vi "SLSC Error Suppression.vi"(3 "error in (no error)":errorcluster, 4 "Popup Error?":bool, 5 "Clear All Error?":bool) -> (6 "error?":bool, 10 "error out":errorcluster)   [LabVIEW 2015, in "SLSC CD Shared.lvlib"]
uses:
  SLSC CD Shared.lvlib
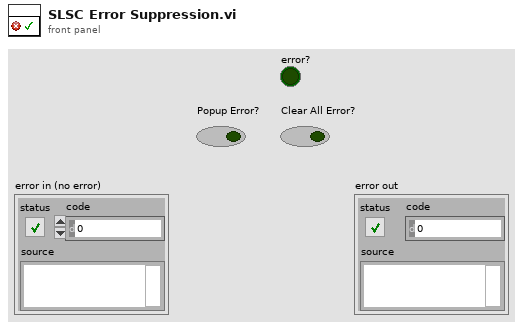
[diagram p1: front panel]
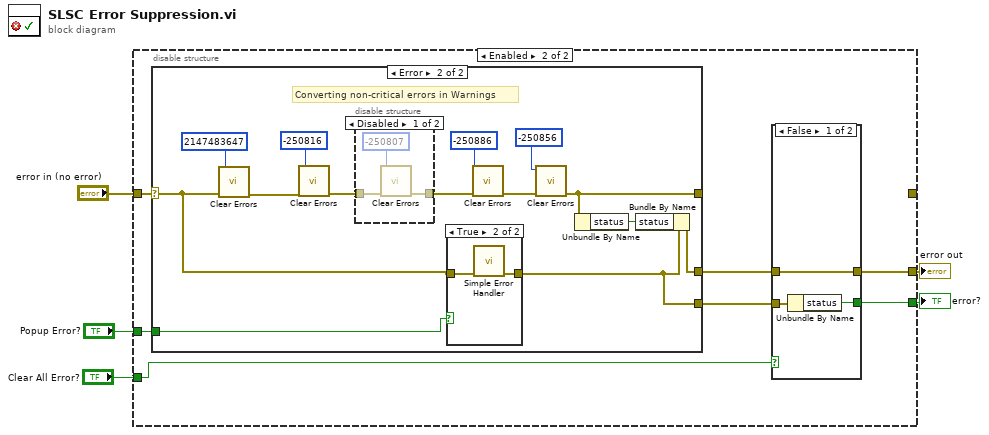
[diagram p0: block diagram]
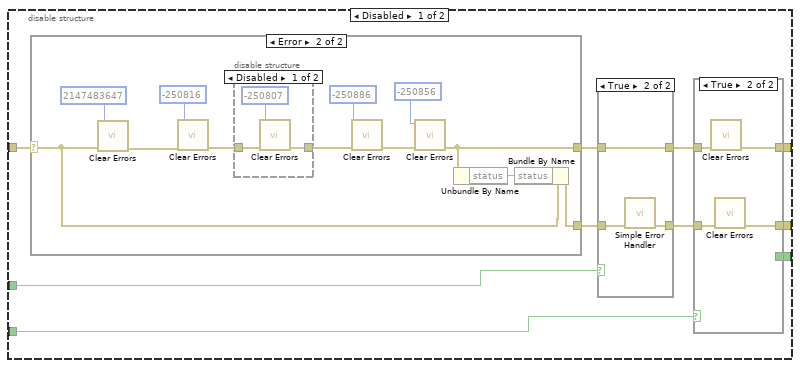
[diagram p2: hidden frame]
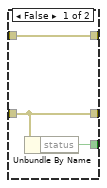
[diagram p3: hidden frame]
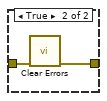
[diagram p7: hidden frame]
diagram:
  n1 = disable-structure shown="Enabled" {
    disable-tunnel: "error in (no error)" -> [w15 w51]
    disable-tunnel: "Popup Error?" -> [w14 w46]
    disable-tunnel: [w12 w49] -> w3
    disable-tunnel: [w9 _] -> _
    disable-tunnel: "Clear All Error?" -> [w8 w47]
    disable-tunnel: [w6 w48] -> w1
    frame Disabled {
      n2 = case shown="Error" w15 {
        selector: w15 -> [w28 w29]
        tunnel: [w28 w32] -> w11
        tunnel: [w28 w30] -> w7
        frame No Error {
        }
        frame Error {
          n3 = call <vilib>:"Clear Errors.vi"("error in (no error)"=w29, "specific error code to clear (0: all)"=2147483647) -> ("error out"=w33:errorcluster)  [unwired: 4 in, 1 out]
          n4 = call <vilib>:"Clear Errors.vi"("error in (no error)"=w33, "specific error code to clear (0: all)"=-250816) -> ("error out"=w39:errorcluster)  [unwired: 4 in, 1 out]
          n5 = disable-structure shown="Disabled" {
            disable-tunnel: w39 -> [w42 w44]
            disable-tunnel: [w41 w44] -> w40
            frame Disabled {
              n6 = call <vilib>:"Clear Errors.vi"("error in (no error)"=w42, "specific error code to clear (0: all)"=-250807) -> ("error out"=w41:errorcluster)  [unwired: 4 in, 1 out]
            }
            frame Enabled {
            }
          }
          n7 = call <vilib>:"Clear Errors.vi"("error in (no error)"=w40, "specific error code to clear (0: all)"=-250886) -> ("error out"=w36:errorcluster)  [unwired: 4 in, 1 out]
          n8 = call <vilib>:"Clear Errors.vi"("error in (no error)"=w36, "specific error code to clear (0: all)"=-250856) -> ("error out"=w32:errorcluster)  [unwired: 4 in, 1 out]
          n9 = Unbundle By Name(w32) -> ("status"=w31:bool)
          n10 = Bundle By Name(cluster=w29, "status"=w31) -> (w30:errorcluster)
        }
      }
      n11 = case shown="True" w14 {
        tunnel: w7 -> [w24 w27]
        tunnel: [w24 w26] -> w13
        tunnel: [w23 w25] -> w10
        tunnel: w11 -> [w23 w25]
        frame False {
        }
        frame True {
          n12 = call <vilib>:"Simple Error Handler.vi"("error in (no error)"=w27) -> ("error out"=w26:errorcluster)  [unwired: 4 in, 4 out]
        }
      }
      n13 = case shown="True" w8 {
        tunnel: w13 -> [w17 w22]
        tunnel: [w17 w21] -> w12
        tunnel: w10 -> [w18 w20]
        tunnel: [w18 w19] -> w9
        tunnel: [w16 _] -> w6
        frame False {
          n14 = Unbundle By Name(w17) -> ("status"=w16:bool)
        }
        frame True {
          n15 = call <vilib>:"Clear Errors.vi"("error in (no error)"=w20) -> ("error out"=w19:errorcluster)  [unwired: 5 in, 1 out]
          n16 = call <vilib>:"Clear Errors.vi"("error in (no error)"=w22) -> ("error out"=w21:errorcluster)  [unwired: 5 in, 1 out]
        }
      }
    }
    frame Enabled {
      n17 = case shown="Error" w51 {
        selector: w51 -> [w57 w60]
        tunnel: [w57 w63] -> _
        tunnel: [w57 w61] -> w50
        tunnel: w46 -> [_ w59]
        tunnel: [w57 w58] -> w45
        frame No Error {
        }
        frame Error {
          # "Converting non-critical errors in Warnings"
          n18 = call <vilib>:"Clear Errors.vi"("error in (no error)"=w60, "specific error code to clear (0: all)"=2147483647) -> ("error out"=w64:errorcluster)  [unwired: 4 in, 1 out]
          n19 = call <vilib>:"Clear Errors.vi"("error in (no error)"=w64, "specific error code to clear (0: all)"=-250816) -> ("error out"=w70:errorcluster)  [unwired: 4 in, 1 out]
          n20 = disable-structure shown="Disabled" {
            disable-tunnel: w70 -> [w76 w78]
            disable-tunnel: [w75 w78] -> w71
            frame Disabled {
              n21 = call <vilib>:"Clear Errors.vi"("error in (no error)"=w76, "specific error code to clear (0: all)"=-250807) -> ("error out"=w75:errorcluster)  [unwired: 4 in, 1 out]
            }
            frame Enabled {
            }
          }
          n22 = case shown="True" w59 {
            tunnel: w60 -> [w72 w74]
            tunnel: [w72 w73] -> w58
            frame False {
            }
            frame True {
              n23 = call <vilib>:"Simple Error Handler.vi"("error in (no error)"=w74) -> ("error out"=w73:errorcluster)  [unwired: 4 in, 4 out]
            }
          }
          n24 = call <vilib>:"Clear Errors.vi"("error in (no error)"=w71, "specific error code to clear (0: all)"=-250886) -> ("error out"=w67:errorcluster)  [unwired: 4 in, 1 out]
          n25 = call <vilib>:"Clear Errors.vi"("error in (no error)"=w67, "specific error code to clear (0: all)"=-250856) -> ("error out"=w63:errorcluster)  [unwired: 4 in, 1 out]
          n26 = Unbundle By Name(w63) -> ("status"=w62:bool)
          n27 = Bundle By Name(cluster=w58, "status"=w62) -> (w61:errorcluster)
        }
      }
      n28 = case shown="False" w47 {
        tunnel: w50 -> [w54 w56]
        tunnel: [w54 w55] -> w49
        tunnel: [w53 _] -> w48
        tunnel: w45 -> [w52 _]
        frame False {
          n29 = Unbundle By Name(w52) -> ("status"=w53:bool)
        }
        frame True {
          n30 = call <vilib>:"Clear Errors.vi"("error in (no error)"=w56) -> ("error out"=w55:errorcluster)  [unwired: 5 in, 1 out]
        }
      }
    }
  }
  "error out" <- w3
  "error?" <- w1
